vi "onListenForNewConnection.vi"(8 "error in (no error)":errorcluster, 9 "timeout (ms)":i32=1, 11 "Listener":refnum<class "LocalQueueConnection.lvclass">) -> (0 "error out":errorcluster, 1 "New connection":bool, 2 "timed out":bool, 3 "New Connection":refnum<class "Connection.lvclass">)   [LabVIEW 2013, in "MQTT_Queue.lvlib" / "LocalQueueConnection.lvclass"]
uses:
  LocalQueueConnection.lvclass
  <vilib>/LabVIEW Open Source Project/Connection/Connection/Connection.lvclass
  LocalQueueConnection.lvclass/LocalQueueConnection.ctl
  <vilib>/Utility/error.llb/Error Cluster From Error Code.vi
  <vilib>/ErrorRing/Error Ring.xnode
  <vilib>/LabVIEW Open Source Project/Unicity/RandomStringGenerator/RandomStringGenerator.lvclass
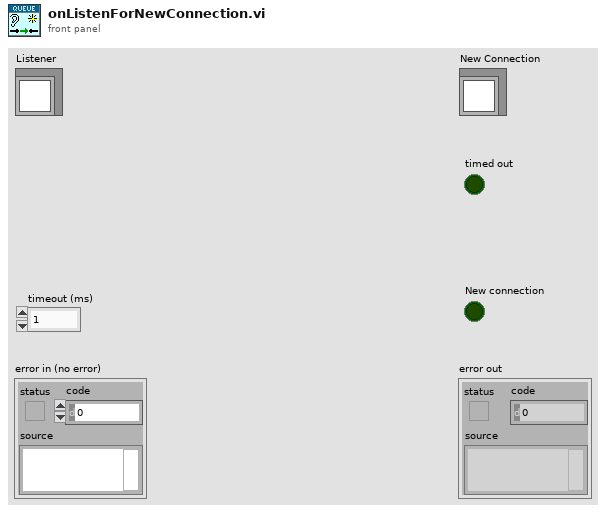
[diagram p1: front panel]
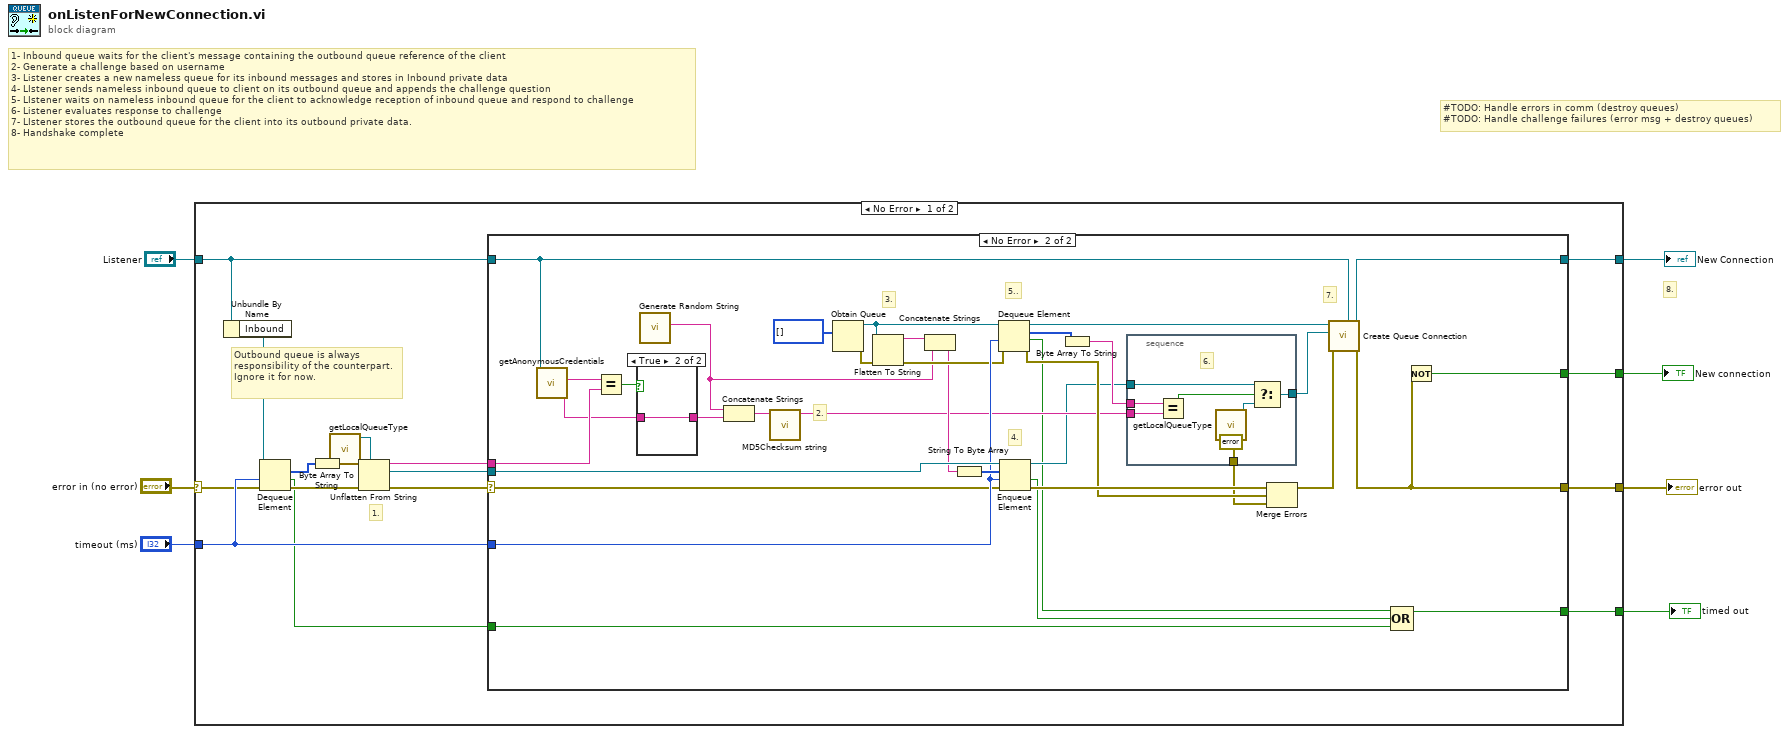
[diagram p0: block diagram]
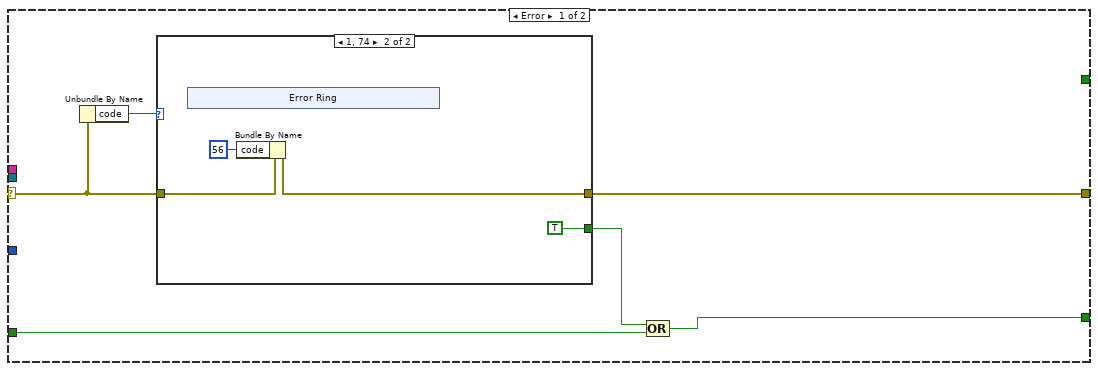
[diagram p2: hidden frame]
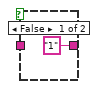
[diagram p4: hidden frame]
diagram:
  # "#TODO: Handle errors in comm (destroy queues)\n#TODO: Handle challenge failures (error msg + destroy queues)"
  # "8."
  # "1- Inbound queue waits for the client's message containing the outbound queue reference of the client\n2- Generate a challenge based on username\n3- Listener creates a new nameless queue for its inbound messages and stores in Inbound private data\n4- LIstener sends nameless inbound queue to client on its outbound queue and appends the challenge question\n5- LIstener waits on nameless inbound queue for the client to acknowledge reception of inbound queue and respond to challenge\n6- Listener evaluates response to challenge\n7- LIstener stores the outbound queue for the client into its outbound private data.\n8- Handshake complete"
  n1 = case shown="No Error" "error in (no error)" {
    selector: "error in (no error)" -> [w8 w83]
    tunnel: [w23 _] -> w7
    tunnel: "timeout (ms)" -> [w17 _]
    tunnel: [w16 w83] -> w5
    tunnel: [w14 _] -> w4
    tunnel: [w12 _] -> w3
    tunnel: "Listener" -> [w10 _]
    frame No Error {
      # "Outbound queue is always responsibility of the counterpart. Ignore it for now."
      # "1."
      n2 = Unbundle By Name(w10) -> ("Inbound"=w21:refnum<queue>)
      n3 = Dequeue Element(queue=w21, timeout in ms (-1)=w17, error in (no error)=w8) -> (element=w22:u8[], timed out?=w11:bool, error out=w19:errorcluster)  [unwired: 1 out]
      n4 = Byte Array To String(unsigned byte array=w22) -> (string=w20:string)
      n5 = call "getLocalQueueType.vi"() -> ("Queue Type"=w15:refnum<queue>)  [unwired: 11 in]
      n6 = Unflatten From String(type=w15, binary string=w20, error in (no error)=w19) -> (rest of the binary string=w13:string, value=w18:refnum<queue>, error out=w9:errorcluster)  [unwired: 2 in]
      n7 = case shown="No Error" w9 {
        selector: w9 -> [w28 w39]
        tunnel: [_ w73] -> w23
        tunnel: w18 -> [_ w69]
        tunnel: w17 -> [_ w67]
        tunnel: [w27 w65] -> w16
        tunnel: [_ w56] -> w14
        tunnel: w13 -> [_ w52]
        tunnel: [w25 w44] -> w12
        tunnel: w11 -> [w26 w41]
        tunnel: w10 -> [_ w40]
        frame Error {
          n8 = Unbundle By Name(w28) -> ("code"=w29:i32)
          n9 = case shown="1, 74" w29 {
            tunnel: w28 -> [w30 w34]
            tunnel: [w30 w32] -> w27
            tunnel: [_ TRUE] -> w24
            frame Default {
            }
            frame 1, 74 {
              n10 = xnode "Error Ring"() -> ()  [unwired: 1 out]
              n11 = Bundle By Name(cluster=w34, "code"=56) -> (w32:errorcluster)
            }
          }
          n12 = Compound Arithmetic op=OR(w24, w26) -> (w25:bool)
        }
        frame No Error {
          # "2."
          # "3."
          # "7."
          # "5.."
          # "4."
          n13 = call "getAnonymousCredentials.vi"("LocalQueueConnection"=w40) -> ("Anonymous password"=w48:string, "Anonymous username"=w55:string)  [unwired: 9 in]
          n14 = Equal?(x=w55, y=w52) -> (x = y?=w50:bool)
          n15 = case shown="True" w50 {
            tunnel: ["1" ("Anonymous password") w75] -> w49
            tunnel: w48 -> [_ w75]
            frame False {
            }
            frame True {
            }
          }
          n16 = call <vilib>:"Generate Random String.vi"() -> ("Random String"=w51:string)  [unwired: 11 in]
          n17 = Concatenate Strings(w51, w49) -> (w54:string)
          n18 = call <vilib>:"MD5Checksum string.vi"("Message String"=w54) -> ("MD5 message-digest"=w53:string)  [unwired: 10 in]
          n19 = Obtain Queue(element data type=u8[] [] ("element")) -> (queue out=w64:refnum<queue>, error out=w63:errorcluster)  [unwired: 4 in, 1 out]
          n20 = Flatten To String(anything=w64, error in (no error)=w63) -> (data string=w60:string, error out=w62:errorcluster)  [unwired: 2 in, 1 out]
          n21 = Concatenate Strings(w60, w51) -> (w57:string)
          n22 = String To Byte Array(string=w57) -> (unsigned byte array=w72:u8[])
          n23 = Dequeue Element(queue=w64, timeout in ms (-1)=w67, error in (no error)=w62) -> (queue out=w68:refnum<queue>, element=w59:u8[], timed out?=w43:bool, error out=w61:errorcluster)
          n24 = Enqueue Element(queue=w69, element=w72, timeout in ms (-1)=w67, error in (no error)=w39) -> (queue out=w46:refnum<queue>, timed out?=w42:bool, error out=w71:errorcluster)
          n25 = Byte Array To String(unsigned byte array=w59) -> (string=w58:string)
          n26 = stacked-sequence {
            tunnel: w58 -> [w81]
            tunnel: w53 -> [w82]
            tunnel: [errorcluster {"status"=FALSE, "code"=0, "source"=""} ("error in")] -> w47
            tunnel: w46 -> [w79]
            tunnel: [w78] -> w45
            frame #0 {
              # "6."
              n27 = Equal?(x=w81, y=w82) -> (x = y?=w77:bool)
              n28 = call "getLocalQueueType.vi"() -> ("Queue Type"=w76:refnum<queue>)  [unwired: 11 in]
              n29 = Select(t=w79, s=w77, f=w76) -> (s? t:f=w78:refnum<queue>)
            }
          }
          n30 = Merge Errors(w71, w61, w47) -> (w66:errorcluster)
          n31 = call "Create Queue Connection.vi"("LocalQueueConnection in"=w40, "error in (no error)"=w66, "Outbound"=w45, "Inbound"=w68) -> ("error out"=w65:errorcluster, "LocalQueueConnection"=w56:refnum<class "LocalQueueConnection.lvclass">)  [unwired: 6 in]
          n32 = Compound Arithmetic op=OR(w43, w42, w41) -> (w44:bool)
          n33 = Not(x=w65) -> (.not. x?=w73:bool)
        }
      }
    }
    frame Error {
    }
  }
  "error out" <- w5
  "New Connection" <- w4
  "New connection" <- w7
  "timed out" <- w3
